vi "MotorControl_MainVI.vi"() -> ()   [LabVIEW 2020]
uses:
  Controls/Main State Machine States.ctl
panel:
  in  "?":refnum<k7>(container)
  out "Angle Serial Number":i32=40808764
  out "States":T1
  out "Progress":u16(slide) scale=0.0..4.0
  in  "?":bool
  in  "Y Axis Step Size":i32
  in  "Y Axis Range":i32
  in  "X Axis Step Size":i32
  in  "X Axis Range":i32
  in  "Angle Step Size":i32
  in  "Angle Range":i32
  in  "?":refnum<k7>(container)
  out "X Translation Serial Number":i32=40849496
  # "Translation Motor"
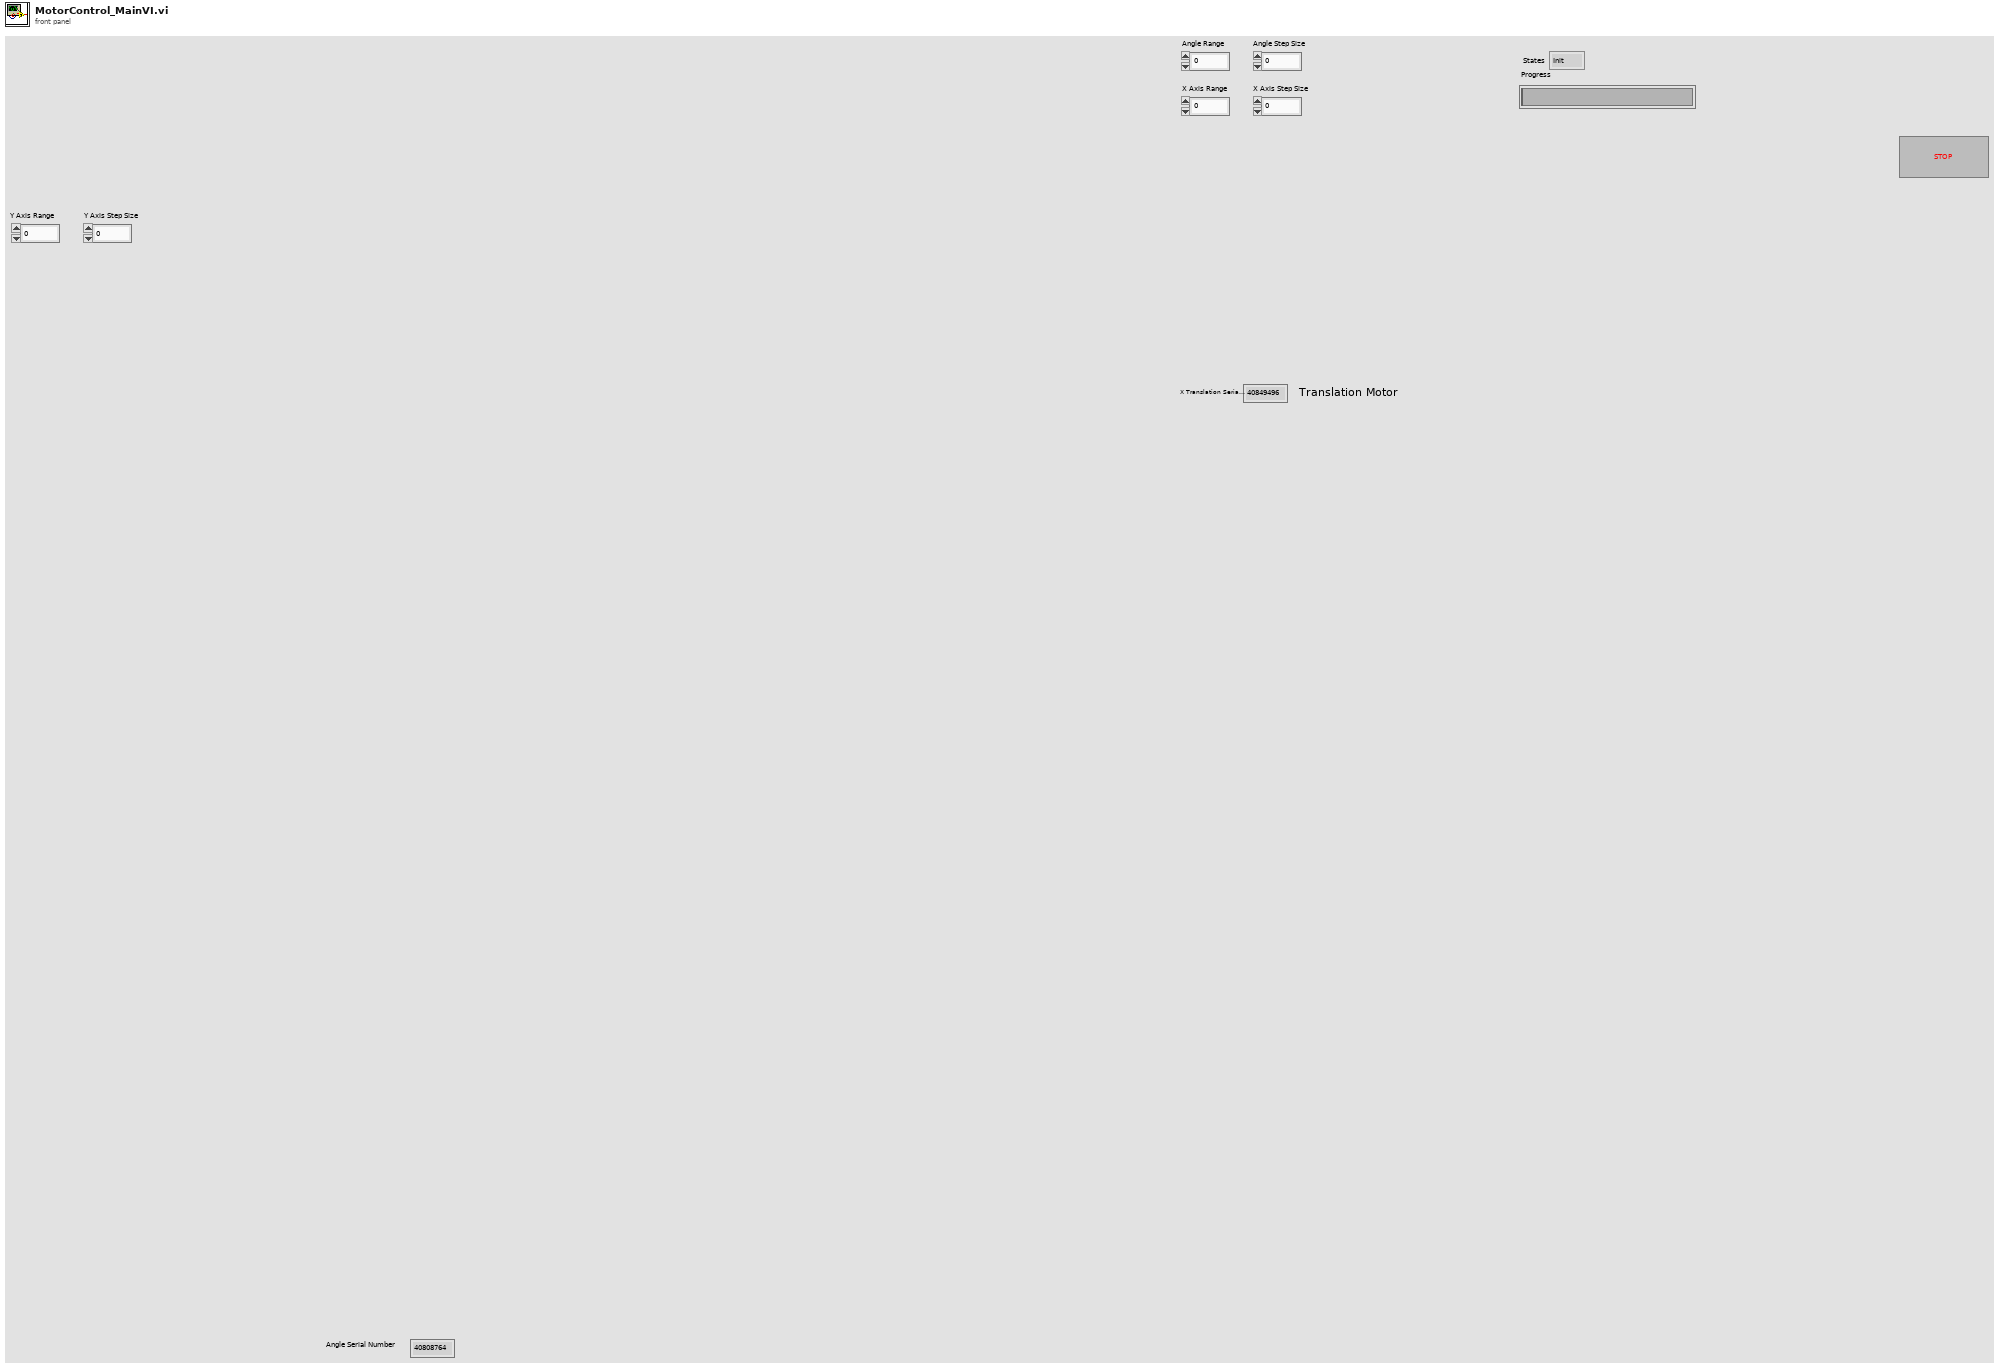
[diagram p1: front panel]
types:
  T1 = typedef "Main State Machine States.ctl" = enum16{"Init", "Theta-Axis Homing", "X-Axis Homing", "Y-axis Homing", "Scanning", "Stop"}
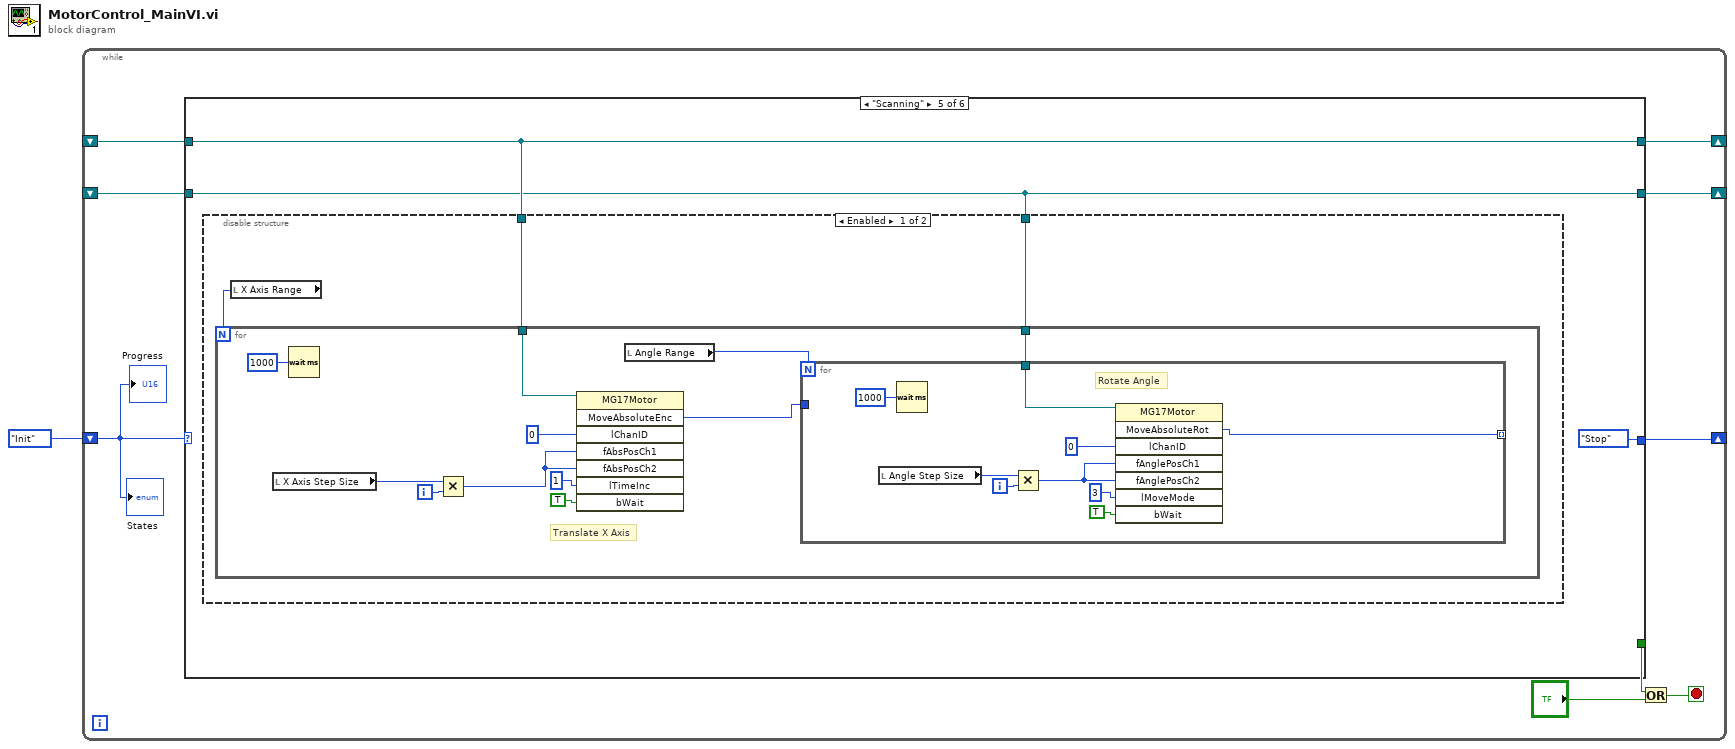
[diagram p0: block diagram]
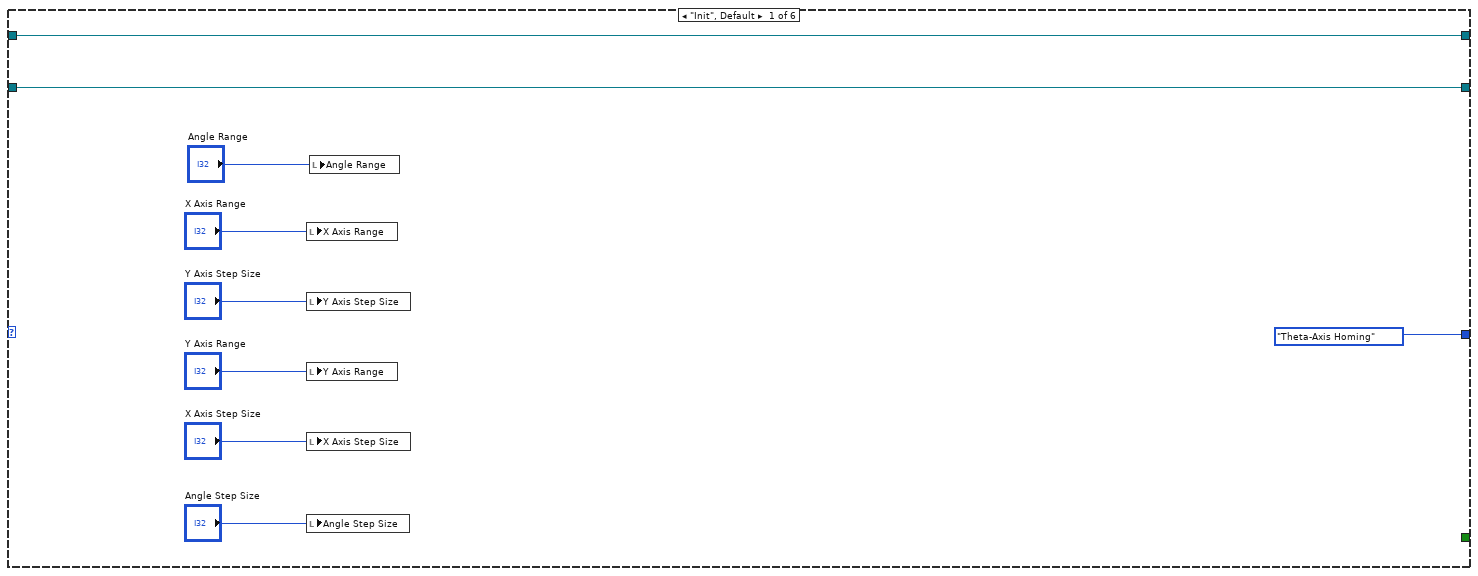
[diagram p2: hidden frame]
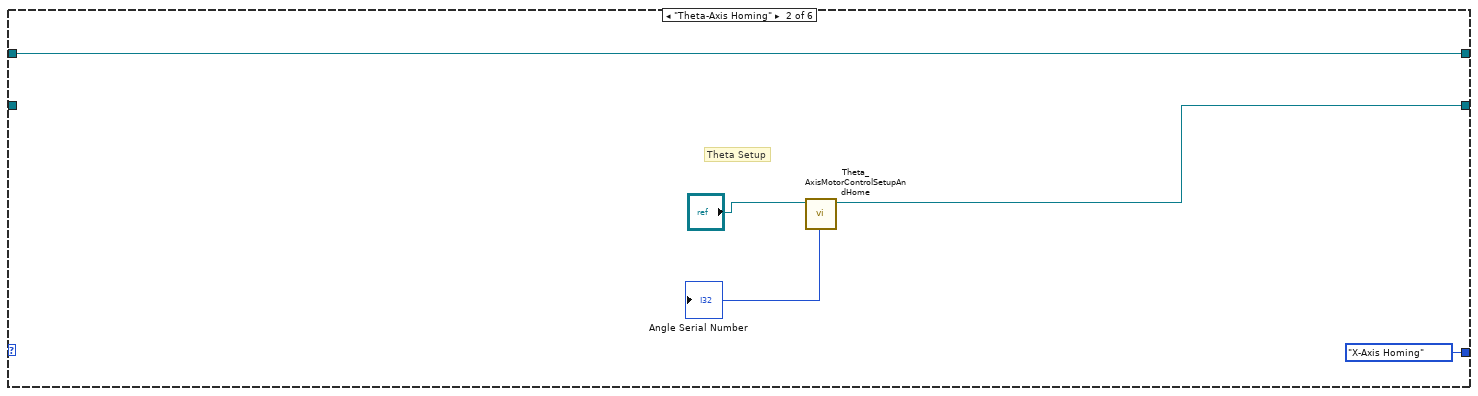
[diagram p3: hidden frame]
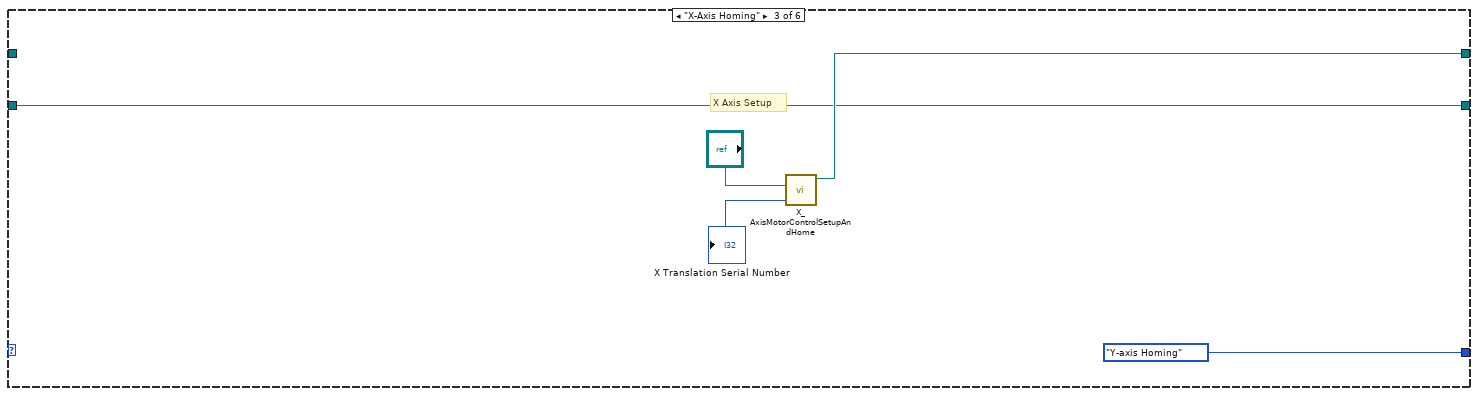
[diagram p4: hidden frame]
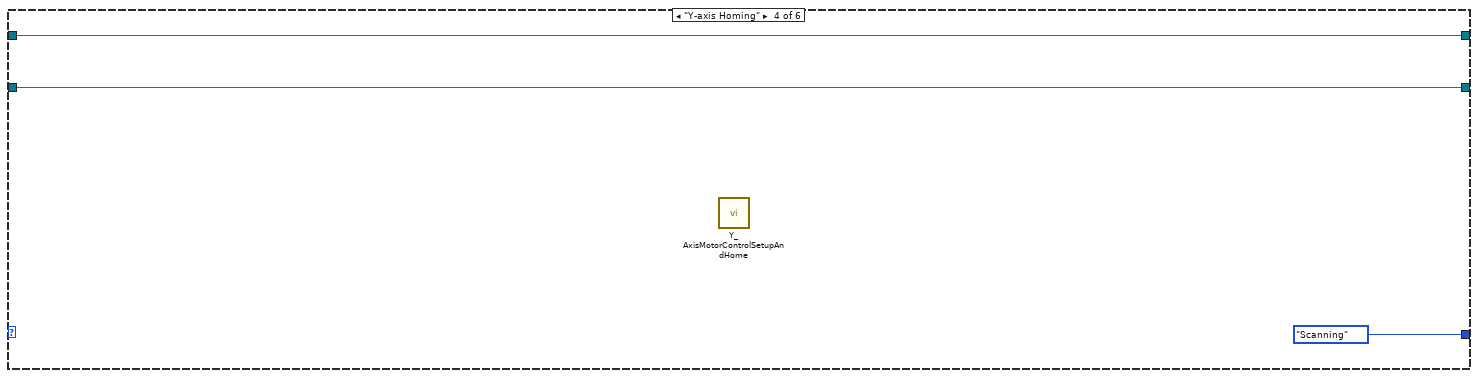
[diagram p5: hidden frame]
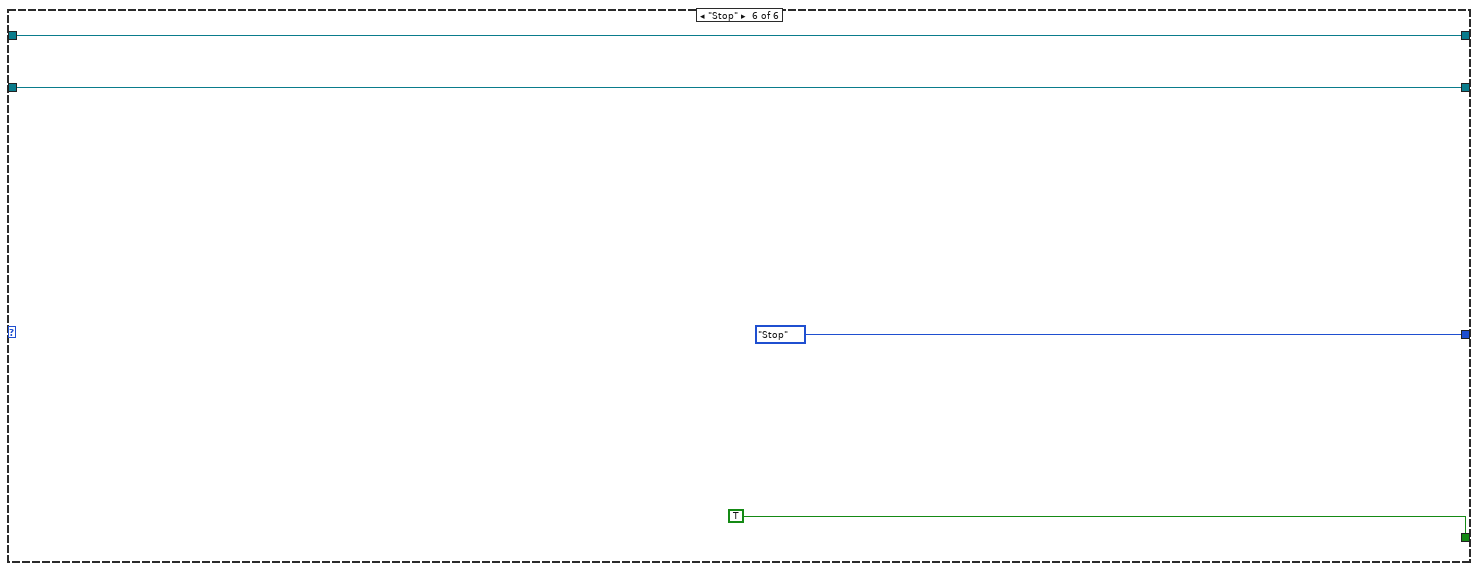
[diagram p7: hidden frame]
diagram:
  n1 = while {
    shift-right: [w10] -> _
    shift-left: Main_State_Machine_States."Init" ("States") -> [w5]
    shift-right: [w9] -> _
    shift-left: _ -> [w8]
    shift-right: [w4] -> _
    shift-left: _ -> [w3]
    stop <- w2 stop-if-true
    n2 = case shown="\"Scanning\"" w5 {
      tunnel: [Main_State_Machine_States."Theta-Axis Homing" ("States") Main_State_Machine_States."X-Axis Homing" ("States") Main_State_Machine_States."Y-axis Homing" ("States") Main_State_Machine_States."Scanning" ("States") Main_State_Machine_States."Stop" ("States") Main_State_Machine_States."Stop" ("States")] -> w10
      tunnel: [w12 w24 w27 w32 w34 w62] -> w9
      tunnel: w8 -> [w12 w24 _ w32 w34 w62]
      tunnel: [_ _ _ _ _ TRUE] -> w7
      tunnel: [w11 w21 w25 w30 w33 w59] -> w4
      tunnel: w3 -> [w11 _ w25 w30 w33 w59]
      frame "Init", Default {
        n3 = local write "X Axis Range"("X Axis Range") -> ()
        n4 = local write "Y Axis Step Size"("Y Axis Step Size") -> ()
        n5 = local write "Y Axis Range"("Y Axis Range") -> ()
        n6 = local write "X Axis Step Size"("X Axis Step Size") -> ()
        n7 = local write "Angle Step Size"("Angle Step Size") -> ()
        n8 = local write "Angle Range"("Angle Range") -> ()
      }
      frame "Theta-Axis Homing" {
        # "Theta Setup"
        n9 = call "Theta_AxisMotorControlSetupAndHome.vi"("Automation Refnum in"="?") -> ("Angle Serial Number"=→"Angle Serial Number":i32, "Automation Refnum out"=w21:refnum<k7>)  [unwired: 9 in]
      }
      frame "X-Axis Homing" {
        # "X Axis Setup"
        n10 = call "X_AxisMotorControlSetupAndHome.vi"("Automation Refnum in"="?") -> ("X Translation Serial Number"=→"X Translation Serial Number":i32, "Automation Refnum out"=w27:refnum<k7>)  [unwired: 9 in]
      }
      frame "Y-axis Homing" {
        n11 = call "Y_AxisMotorControlSetupAndHome.vi"() -> ()  [unwired: 12 in]
      }
      frame "Scanning" {
        n12 = disable-structure shown="Enabled" {
          disable-tunnel: w34 -> [w37 _]
          disable-tunnel: w33 -> [w36 _]
          frame Enabled {
            n13 = local read "X Axis Range"() -> (w38:i32)
            n14 = for {
              N: w38 -> [_]
              tunnel: w37 -> [w40]
              tunnel: w36 -> [w39]
              i -> [w44]
              # "Translate X Axis"
              n15 = local read "X Axis Step Size"() -> (w46:i32)
              n16 = Wait (ms)(milliseconds to wait=u32 1000) -> ()  [unwired: 1 out]
              n17 = Multiply(x=w46, y=w44) -> (x*y=w45:i32)
              n18 = invoke class="MG17Motor" method="MoveAbsoluteEnc"(reference=w40, "lChanID"=0, "fAbsPosCh1"=w45, "fAbsPosCh2"=w45, "lTimeInc"=1, "bWait"=TRUE) -> ("MoveAbsoluteEnc"=w41:i32)  [unwired: 2 in, 7 out]
              n19 = local read "Angle Range"() -> (w42:i32)
              n20 = for {
                N: w42 -> [_]
                tunnel: w41 -> [_]
                tunnel: [w51] -> _ mode=indexing
                tunnel: w39 -> [w50]
                i -> [w53]
                # "Rotate Angle"
                n21 = local read "Angle Step Size"() -> (w55:i32)
                n22 = Wait (ms)(milliseconds to wait=u32 1000) -> ()  [unwired: 1 out]
                n23 = Multiply(x=w55, y=w53) -> (x*y=w54:i32)
                n24 = invoke class="MG17Motor" method="MoveAbsoluteRot"(reference=w50, "lChanID"=0, "fAnglePosCh1"=w54, "fAnglePosCh2"=w54, "lMoveMode"=3 ("lTimeInc"), "bWait"=TRUE) -> ("MoveAbsoluteRot"=w51:i32)  [unwired: 2 in, 7 out]
              }
            }
          }
          frame Disabled {
          }
        }
      }
      frame "Stop" {
      }
    }
    n25 = Or(x=w7, y="?") -> (x .or. y?=w2:bool)
    "Progress" <- w5
    "States" <- w5
  }
